vi "x = y (+-epsilon) [DBL].vi"(2 "epsilon (machine)":dbl=2.220446049250313e-16, 5 "x":dbl, 9 "y":dbl) -> (8 "x = y +/- epsilon":bool)   [LabVIEW 2021, in "Comparison.lvlib"]
uses:
  Comparison.lvlib
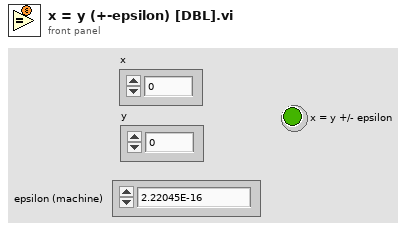
[diagram p1: front panel]
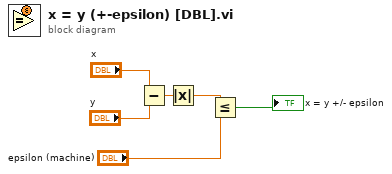
[diagram p0: block diagram]
diagram:
  n1 = Subtract(x="x", y="y") -> (x-y=w4:dbl)
  n2 = Absolute Value(x=w4) -> (abs(x)=w3:dbl)
  n3 = Less Or Equal?(x=w3, y="epsilon (machine)") -> (x <= y?=→"x = y +/- epsilon":bool)
